vi "Write to File.vi"(8 "error in (no error)":errorcluster, 10 "INI Ref":T1, 11 "Timing Action in":refnum<class "Timing Action.lvclass">) -> (0 "error out":errorcluster, 2 "INI Ref out":T1, 3 "Timing Action out":refnum<class "Timing Action.lvclass">)   [LabVIEW 2020, in "MacroAssert.lvlib" / "Timing Action.lvclass"]
uses:
  Timing Action.lvclass
  Action Step/Action Step.lvclass
  Timing Action.lvclass/Timing Action.ctl
  MacroAssert.lvlib
  <vilib>/Utility/config.llb/NI_LVConfig.lvlib
  <vilib>/Utility/config.llb/Write Key (String).vi
  <vilib>/Utility/config.llb/Write Key (Double).vi
  <vilib>/Utility/config.llb/Config Data RefNum.ctl
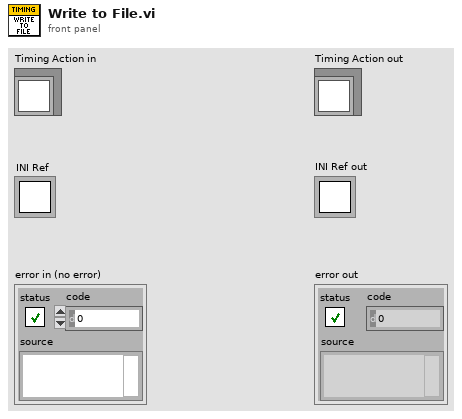
[diagram p1: front panel]
types:
  T1 = typedef "NI_LVConfig.lvlib/Config Data RefNum.ctl" = refnum<k1>
  T2 = typedef "MacroAssert.lvlib/Timing Action.lvclass/Timing Action Type.ctl" = enum16{"Wait", "Wait Until"}
  T3 = typedef "MacroAssert.lvlib/Timing Action.lvclass/Time Unit.ctl" = enum16{"milliseconds", "seconds", "minutes"}
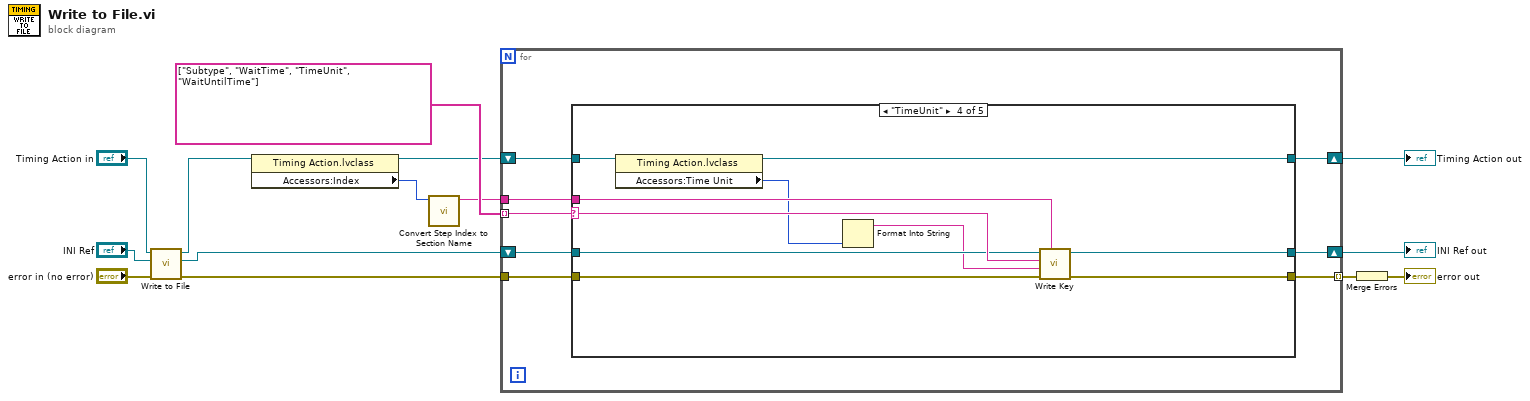
[diagram p0: block diagram]
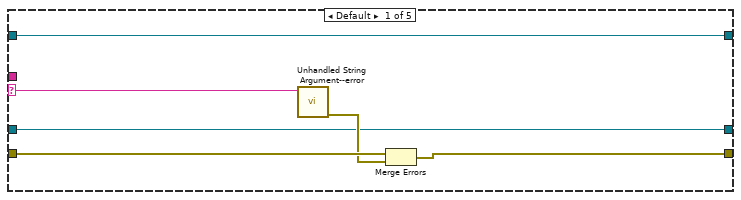
[diagram p2: hidden frame]
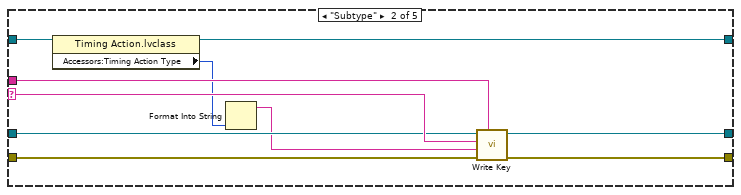
[diagram p3: hidden frame]
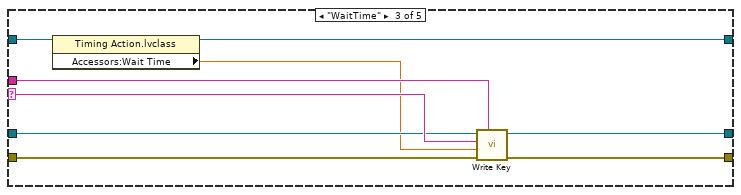
[diagram p4: hidden frame]
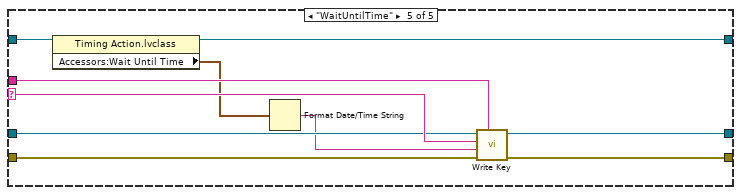
[diagram p5: hidden frame]
diagram:
  n1 = call-parent "Write to File.vi"("error in (no error)"="error in (no error)", "INI Ref"="INI Ref", "Step in"="Timing Action in") -> ("error out"=w9:errorcluster, "INI Ref out"=w7:T1, "Step out"=w8:refnum<class "Timing Action.lvclass">)  [unwired: 6 in]
  n2 = property class="Timing Action.lvclass"(reference=w8) -> (reference out=w11:refnum<class "Timing Action.lvclass">, "Accessors:Index"=w14:i32)  [unwired: 1 in, 1 out]
  n3 = call "Convert Step Index to Section Name.vi"("Step Index"=w14) -> ("Section Name"=w10:string)  [unwired: 10 in]
  n4 = for {
    tunnel: string[] ["Subtype", "WaitTime", "TimeUnit", "WaitUntilTime"] -> [w22] mode=indexing
    tunnel: w9 -> [w21]
    tunnel: w10 -> [w20]
    shift-right: [w18] -> w1
    shift-left: w11 -> [w19]
    tunnel: [w17] -> w12 mode=indexing
    shift-right: [w15] -> w2
    shift-left: w7 -> [w16]
    n5 = case shown="\"TimeUnit\"" w22 {
      selector: w22 -> [w25 w36 w45 w55 w65]
      tunnel: w21 -> [w27 w38 w47 w57 w67]
      tunnel: w20 -> [_ w37 w46 w56 w66]
      tunnel: w19 -> [w28 w34 w43 w53 w63]
      tunnel: [w28 w29 w40 w50 w60] -> w18
      tunnel: [w24 w33 w42 w52 w62] -> w17
      tunnel: w16 -> [w23 w35 w44 w54 w64]
      tunnel: [w23 w32 w41 w51 w61] -> w15
      frame Default {
        n6 = call "Unhandled String Argument--error.vi"("Argument"=w25) -> ("error out"=w26:errorcluster)  [unwired: 10 in]
        n7 = Merge Errors(w27, w26) -> (w24:errorcluster)
      }
      frame "Subtype" {
        n8 = property class="Timing Action.lvclass"(reference=w34) -> (reference out=w29:refnum<class "Timing Action.lvclass">, "Accessors:Timing Action Type"=w31:T2)  [unwired: 1 in, 1 out]
        n9 = Format Into String(w31) -> (resulting string=w30:string)  [unwired: 3 in, 1 out]
        n10 = call-poly <vilib>:"Write Key.vi"("section"=w37, "error in (no error)"=w38, "value"=w30, "key"=w36, "refnum"=w35) -> ("error out"=w33:errorcluster, "refnum out"=w32:T1)  [unwired: 4 in, 1 out]
      }
      frame "WaitTime" {
        n11 = property class="Timing Action.lvclass"(reference=w43) -> (reference out=w40:refnum<class "Timing Action.lvclass">, "Accessors:Wait Time"=w39:dbl)  [unwired: 1 in, 1 out]
        n12 = call-poly <vilib>:"Write Key.vi"("section"=w46, "error in (no error)"=w47, "value"=w39, "key"=w45, "refnum"=w44) -> ("error out"=w42:errorcluster, "refnum out"=w41:T1)  [unwired: 4 in, 1 out]
      }
      frame "TimeUnit" {
        n13 = property class="Timing Action.lvclass"(reference=w53) -> (reference out=w50:refnum<class "Timing Action.lvclass">, "Accessors:Time Unit"=w49:T3)  [unwired: 1 in, 1 out]
        n14 = Format Into String(w49) -> (resulting string=w48:string)  [unwired: 3 in, 1 out]
        n15 = call-poly <vilib>:"Write Key.vi"("section"=w56, "error in (no error)"=w57, "value"=w48, "key"=w55, "refnum"=w54) -> ("error out"=w52:errorcluster, "refnum out"=w51:T1)  [unwired: 4 in, 1 out]
      }
      frame "WaitUntilTime" {
        n16 = property class="Timing Action.lvclass"(reference=w63) -> (reference out=w60:refnum<class "Timing Action.lvclass">, "Accessors:Wait Until Time"=w59:timestamp)  [unwired: 1 in, 1 out]
        n17 = Format Date/Time String(seconds (now)=w59) -> (date/time string=w58:string)  [unwired: 2 in]
        n18 = call-poly <vilib>:"Write Key.vi"("section"=w66, "error in (no error)"=w67, "value"=w58, "key"=w65, "refnum"=w64) -> ("error out"=w62:errorcluster, "refnum out"=w61:T1)  [unwired: 4 in, 1 out]
      }
    }
  }
  "Timing Action out" <- w1
  "INI Ref out" <- w2
  n19 = Merge Errors(w12) -> (→"error out":errorcluster)
